vi "Stop Core.vi"(10 "final error code":i32, 11 "Mag Lab Measure Base in":refnum<class "Mag Lab Measure Base.lvclass">) -> (3 "Mag Lab Measure Base out":refnum<class "Mag Lab Measure Base.lvclass">)   [LabVIEW 2015, in "Mag Lab Measure Base.lvclass"]
doc: "(<B>Filename</B>: Actor Framework.lvlib:Actor.lvclass:Stop Core.vi)\n\nDefines what the actor does before it stops. Use the <B>final error code</B> input to determine whether the actor shut down in response to an error.\n\nBy default, this method does nothing. A descendant class may override it to define behavior, such as shutting down any processes the actor initiated in its override of the Actor Core method."
uses:
  Mag Lab Measure Base.lvclass
  Mag Lab Root/Mag Lab Root.lvclass/Mag Lab Root.ctl
  <vilib>/ActorFramework/Actor/Actor.lvclass/Actor.ctl
  Mag Lab Measure Base.lvclass/Mag Lab Measure Base.ctl
  Mag Lab Measure Base Messages/Nested Object Stopped Msg/Nested Object Stopped Msg.lvclass/Nested Object Stopped Msg.ctl
  <vilib>/ActorFramework/Message Enqueuer/Message Enqueuer.lvclass/Message Enqueuer.ctl
  <vilib>/ActorFramework/Message Enqueuer/Enqueue.vi
  <vilib>/ActorFramework/Message Priority Queue/Priority Enqueue.vi
  Mag Lab Measure Base Messages/Nested Object Stopped Msg/Nested Object Stopped Msg.lvclass
  <vilib>/ActorFramework/Stop Msg/Stop Msg.lvclass
  Mag Lab Root/Mag Lab Root.lvclass
  <vilib>/ActorFramework/Actor/Actor.lvclass
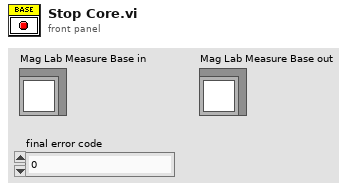
[diagram p1: front panel]
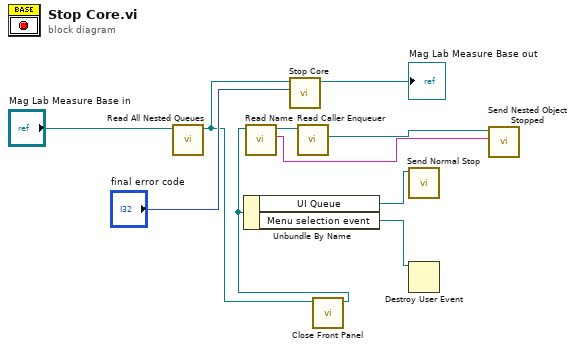
[diagram p0: block diagram]
diagram:
  n1 = call "Read All Nested Queues.vi"("Mag Lab Measure Base in"="Mag Lab Measure Base in") -> ("Mag Lab Measure Base out"=w2:refnum<class "Mag Lab Measure Base.lvclass">)  [unwired: 7 in, 3 out]
  n2 = call-parent "Stop Core.vi"("final error code"="final error code", "Mag Lab Root in"=w2) -> ("Mag Lab Root out"=→"Mag Lab Measure Base out":refnum<class "Mag Lab Measure Base.lvclass">)  [unwired: 9 in]
  n3 = call-dynamic "Close Front Panel.vi"("Mag Lab Root in"=w2) -> ("Mag Lab Root out"=w1:refnum<class "Mag Lab Measure Base.lvclass">)  [unwired: 9 in, 1 out]
  n4 = Unbundle By Name(w1) -> ("UI Queue"=w6:refnum<class "Message Enqueuer.lvclass">, "Menu selection event"=w5:refnum<user-event>)
  n5 = call "Read Name.vi"("Mag Lab Root in"=w1) -> ("Name"=w3:string, "Mag Lab Root out"=w4:refnum<class "Mag Lab Measure Base.lvclass">)  [unwired: 8 in, 1 out]
  n6 = call <vilib>:"Read Caller Enqueuer.vi"("Actor"=w4) -> ("Caller Enqueuer"=w7:refnum<class "Message Enqueuer.lvclass">)  [unwired: 10 in]
  n7 = call <vilib>:"Send Normal Stop.vi"("Message Enqueuer"=w6) -> ()  [unwired: 10 in, 1 out]
  n8 = Destroy User Event(user event=w5) -> ()  [unwired: 1 in, 1 out]
  n9 = call "Send Nested Object Stopped.vi"("Name"=w3, "Message Enqueuer"=w7) -> ()  [unwired: 8 in, 2 out]
